vi "bump_test.vi"() -> ()   [LabVIEW 2017]
uses:
  <vilib>/myRIO/Common/Instrument Driver Framework/myRIO v1.0/UART/vis/myRIO v1.0 Close UART.vi
  <vilib>/myRIO/Common/Instrument Driver Framework/Utilities/vis/FPGA Ref Manager.vi
  <vilib>/myRIO/Common/Instrument Driver Framework/myRIO v1.0/myRIO v1.0 Reset FPGA.vi
  <vilib>/myRIO/Common/Instrument Driver Framework/myRIO v1.0/IRQ/vis/myRIO v1.0 IRQ Info FGV.vi
  <vilib>/myRIO/Common/Instrument Driver Framework/myRIO v1.0/IRQ/vis/myRIO v1.0 Timer IRQ Info FGV.vi
  <vilib>/myRIO/Common/Instrument Driver Framework/myRIO v1.0/IRQ/vis/myRIO v1.0 ISR Agent.vi
  <vilib>/myRIO/Instrument Drivers/Utilities/Utilities.lvlib
panel:
  out "Motion Data":T1
  out "Output String":string
  in  "stop":bool
  in  "Frequency":dbl
  out "dt (s)":dbl format="%.3f"
  out "Speed & Output":T2(graph)
  in  "DC% Output":dbl
  out "Time (s)":dbl
  in  "FWD/RVS":bool
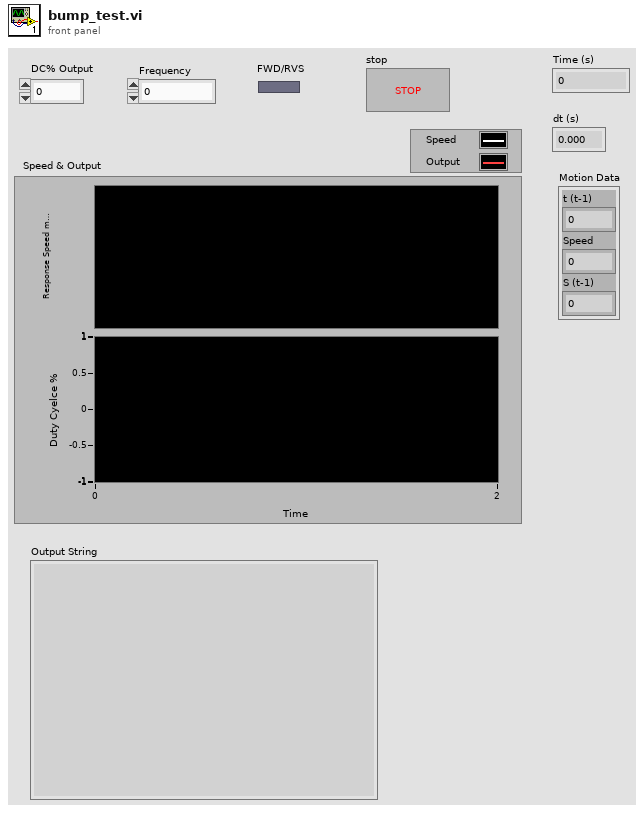
[diagram p1: front panel]
types:
  T1 = cluster{"t (t-1)":u32, "Speed":dbl, "S (t-1)":dbl}
  T2 = cluster{"Velocity Set Pt":dbl, "Velocity (mm/s)":dbl}
  T3 = cluster{"Velocity Set Pt":dbl, "Velocity (mm/s)":dbl}[]
  T4 = typedef "Encoder Cluster.ctl" = cluster{"Y-axis rev count":dbl, "Y-axis distance":dbl, "X-axis rev count":dbl, "X-axis distance":dbl, "Y-axis direction":T5, "X-axis direction":T5, "X-counter val":i32, "Y-counter val":i32}
  T5 = typedef "Encoder Count Direction Enum.ctl" = enum16{"Counting Up", "Counting Down"}
  T6 = cluster{dbl, "Velocity Set Pt":dbl, dbl, "DC% Output":dbl}
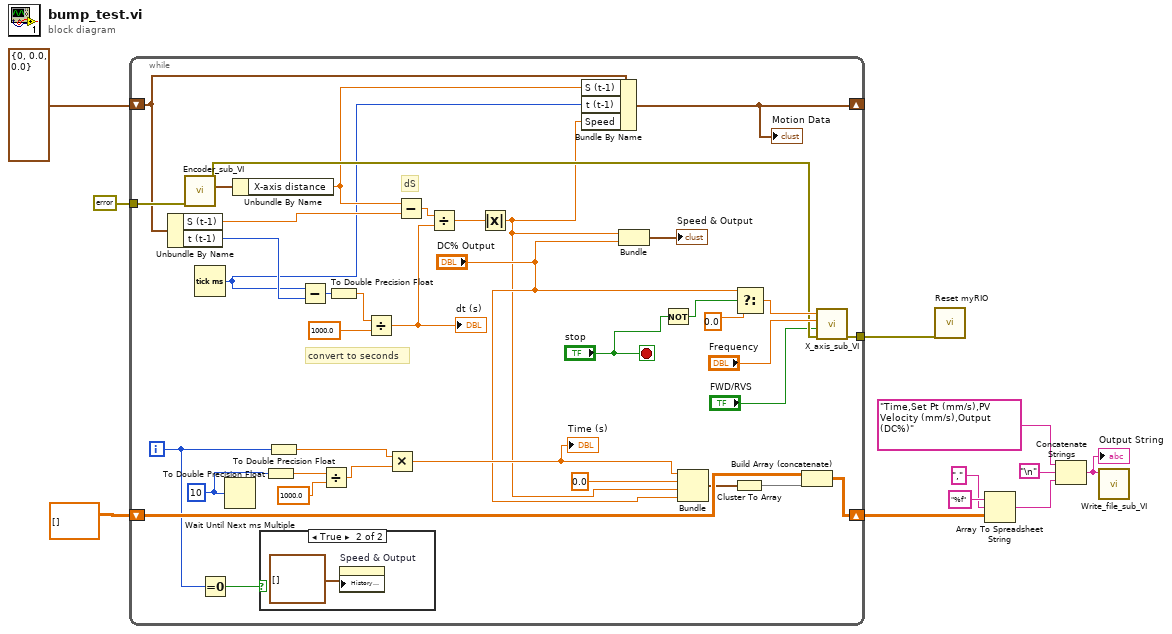
[diagram p0: block diagram]
diagram:
  n1 = while {
    shift-right: [w19] -> w4
    shift-left: dbl[][] [] ("element") -> [w37]
    tunnel: errorcluster {"status"=FALSE, "code"=0, "source"=""} ("error constant") -> [w36]
    tunnel: [w34] -> w2
    shift-right: [w12] -> _
    shift-left: T1 {"t (t-1)"=0, "Speed"=0.0, "S (t-1)"=0.0} ("Motion Data") -> [w17]
    i -> [w25]
    stop <- "stop" stop-if-true
    w28 = u32 10 ("millisecond multiple")
    # "dS"
    # "convert to seconds"
    n2 = Unbundle By Name(w17) -> ("S (t-1)"=w18:dbl, "t (t-1)"=w15:u32)
    n3 = call "Encoder_sub_VI.vi"("error in (no error)"=w36) -> ("error out"=w35:errorcluster, "Encoder Output"=w48:T4)  [unwired: 9 in]
    n4 = Tick Count (ms)() -> (millisecond timer value=w14:u32)
    n5 = Equal To 0?(x=w25) -> (x = 0?=w26:bool)
    n6 = Wait Until Next ms Multiple(millisecond multiple=w28) -> ()  [unwired: 1 out]
    n7 = Unbundle By Name(w48) -> ("X-axis distance"=w16:dbl)
    n8 = case shown="True" w26 {
      frame False {
      }
      frame True {
        n9 = property on="Speed & Output" class="WFChart (strict)"("History Data"=T3 []) -> ()  [unwired: 2 in, 2 out]
      }
    }
    n10 = To Double Precision Float(number=w28) -> (double precision float=w33:dbl)
    n11 = To Double Precision Float(number=w25) -> (double precision float=w29:dbl)
    n12 = Subtract(x=w14, y=w15) -> (x-y=w40:u32)
    n13 = Divide(x=w33, y=1000.0) -> (x/y=w31:dbl)
    n14 = To Double Precision Float(number=w40) -> (double precision float=w39:dbl)
    n15 = Divide(x=w39, y=1000.0) -> (x/y=w38:dbl)
    "dt (s)" <- w38
    n16 = Multiply(x=w29, y=w31) -> (x*y=w30:dbl)
    "Time (s)" <- w30
    n17 = Subtract(x=w16, y=w18) -> (x-y=w47:dbl)
    n18 = Divide(x=w47, y=w38) -> (x/y=w46:dbl)
    n19 = Absolute Value(x=w46) -> (abs(x)=w13:dbl)
    n20 = Bundle By Name(cluster=w17, "S (t-1)"=w16, "t (t-1)"=w14, "Speed"=w13) -> (w12:T1)
    "Motion Data" <- w12
    n21 = Bundle(w13, "DC% Output"="DC% Output") -> (→"Speed & Output":cluster{dbl, "DC% Output":dbl})  [unwired: 1 in]
    n22 = Not(x="stop") -> (.not. x?=w44:bool)
    n23 = Bundle(w30, "Velocity Set Pt"=0.0, w13, "DC% Output"="DC% Output") -> (w21:T6)  [unwired: 1 in]
    n24 = Cluster To Array(cluster=w21) -> (array=w20:dbl[])
    n25 = Select(t="DC% Output", s=w44, f=0.0) -> (s? t:f=w42:dbl)
    n26 = Build Array (concatenate)(w37, w20) -> (w19:dbl[][])
    n27 = call "X_axis_sub_VI.vi"("error in (no error)"=w35, "FWD/RVS"="FWD/RVS", "Frequency"="Frequency", "Duty Cycle %"=w42) -> ("error out"=w34:errorcluster)  [unwired: 7 in]
  }
  n28 = call <vilib>:"Reset myRIO.vi"("error in (no error)"=w2) -> ()  [unwired: 10 in, 1 out]
  n29 = Array To Spreadsheet String(delimiter (Tab)=",", array=w4, 3:"%f" ("format string")) -> (spreadsheet string=w10:string)
  n30 = Concatenate Strings("Time,Set Pt (mm/s),PV Velocity (mm/s),Output (DC%)", "\n", w10) -> (w9:string)
  "Output String" <- w9
  n31 = call "Write_file_sub_VI.vi"("Output String"=w9) -> ()  [unwired: 9 in, 2 out]
